vi "S2C_Globals.vi"() -> ()   [LabVIEW 2024]
panel:
  out "EventStart":dbl
  out "Break?":bool
  out "LastStep?":bool
  out "BOF_Active?":bool
  in  "ExeRetest":refnum<vi>
  out "BreakOnFail?":bool
  out "TestStart":dbl
  out "StepStart":dbl
  in  "QV-Exit":refnum<vi>
  in  "Exit":refnum<vi>
  out "Paused?":bool
  in  "LoopText":refnum<vi>
  in  "LoopMax":i32
  in  "LoopCnt":i32
  in  "ExeLoad":refnum<vi>
  in  "ScriptFile":path
  out "EngLoad?":bool
  out "Aborting?":bool
  in  "Tab":refnum<vi>
  in  "LoopLED":refnum<vi>
  out "Looping?":bool
  in  "SubScriptPath":path
  in  "BldBack":refnum<vi>
  in  "BldSubScr":refnum<vi>
  in  "ReportPath":path
  out "LocalResults":bool
  in  "ExeScrFile":refnum<vi>
  in  "BldScr":refnum<vi>
  in  "ScriptPath":path
  in  "VI Ref":refnum<vi>
  in  "Error":errorcluster
  in  "S2C-Q":refnum<queue>
  out "CustomError":cluster{"Code":i32, "Source":string}[](array[cluster])=[{"Code"=5000, "Source"="The HWT Settings file could not be found.\n\nContact Engineering:  The app will now exit!"}, {"Code"=5005, "Source"="The application was unable to successfully launch Fornax.\n\nContact Engineering:  The app will now exit!"}, {"Code"=6000, "Source"="The requested TouchScreen location was not found in the Settings file."}, {"Code"=6005, "Source"="The requested Insert/Extract instrument was not found in the Settings file."}, {"Code"=6010, "Source"="The requested HandSwitch instrument was not found in the Settings file."}, {"Code"=6015, "Source"="The requested FootSwitch instrument was not found in the Settings file."}, {"Code"=6020, "Source"="The requested Relay Path was not found in the Settings file."}, {"Code"=6025, "Source"="An error occurred attempting to Open a connection to the M4X Analyzer."}, {"Code"=6026, "Source"="An error occurred attempting to Close the connection to the M4X Analyzer."}, {"Code"=6030, "Source"="An error occurred attempting to Open a connection to the Uni-Therm."}, {"Code"=6031, "Source"="The Uni-Therm failed to respond to an identification request."}, {"Code"=6032, "Source"="An error occurred attempting to Set the Uni-Therm load."}, {"Code"=6033, "Source"="An error occurred attempting to Clear the Uni-Therm load."}, {"Code"=6034, "Source"="The Uni-Therm failed to indicate the load has been cleared."}, {"Code"=6053, "Source"="The Uni-Therm failed to indicate the load has been set."}, {"Code"=6040, "Source"="This script contains a configuration name that cound not be found in the Configuration file.\n\nThe script load operation has been aborted!"}]
  in  "ExePause":refnum<vi>
  in  "ExeNext":refnum<vi>
  in  "ExeStart":refnum<vi>
  out "Running?":bool
  in  "ExeScript":string[][](array[string])
  in  "ExeIndex":i32
  in  "ExeTable":refnum<vi>
  in  "BldTable":refnum<vi>
  in  "FPGA_Ref":refnum<k20>
  in  "Settings File":path
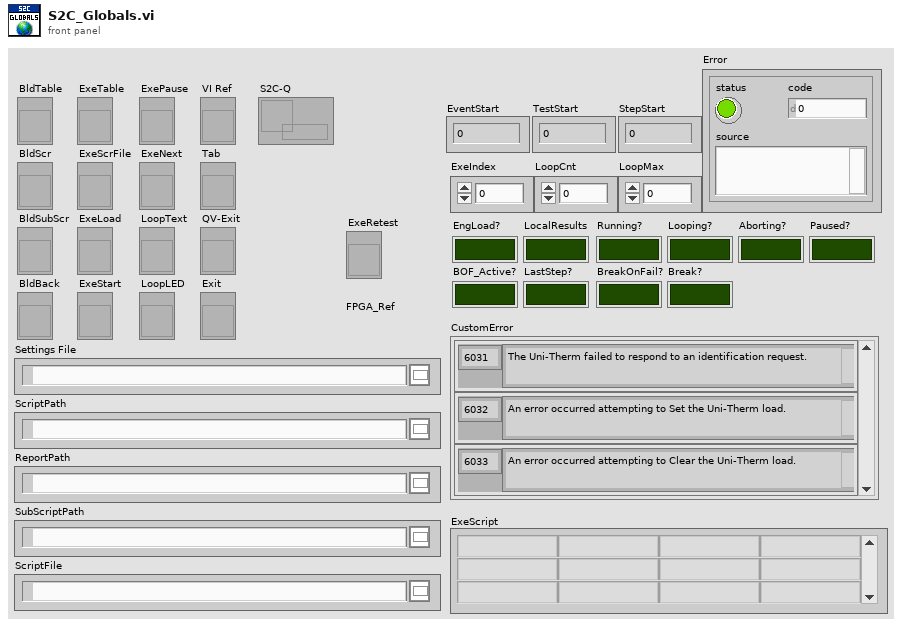
[diagram p1: front panel]
diagram:
